vi "GrabberOPENandCLOSE.vi"(8 "Error In":errorcluster, 9 "Grabber Open/Close":bool, 11 "refnum name":string="My Solenoid RefNum") -> (0 "Error Out":errorcluster)   [LabVIEW 2014]
uses:
  <vilib>/Rock Robotics/WPI/Solenoid/WPI_SolenoidValue.ctl
  <vilib>/Rock Robotics/WPI/Solenoid/WPI_SolenoidSetEnum.vi
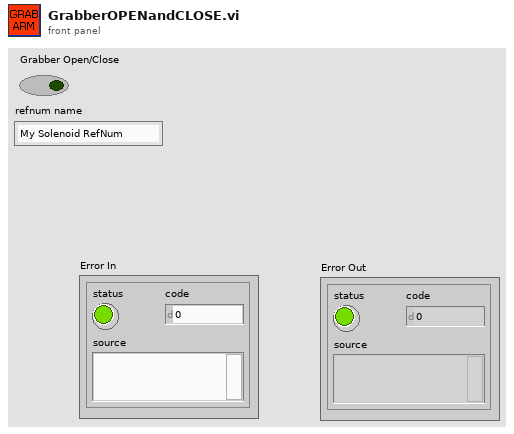
[diagram p1: front panel]
types:
  T1 = typedef "WPI_SolenoidValue.ctl" = enum16{"Off", "On", "Forward", "Reverse"}
  T2 = typedef "WPI_SolenoidDevRef.ctl" = cluster{"DevStatus":errorcluster, "Pneumatics Control Module":u8, "Forward Solenoid Channel":T3, "Reverse Solenoid Channel":T3}
  T3 = typedef "WPI_SolenoidChannel.ctl" = enum8{"Solenoid 0", "Solenoid 1", "Solenoid 2", "Solenoid 3", "Solenoid 4", "Solenoid 5", "Solenoid 6", "Solenoid 7", "Invalid"}
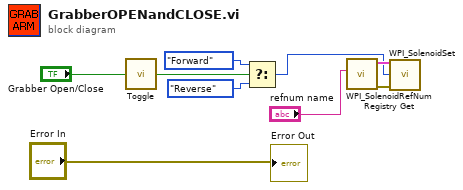
[diagram p0: block diagram]
diagram:
  n1 = call "Toggle.vi"("Input"="Grabber Open/Close") -> ("Output"=w9:bool)
  n2 = Select(t=WPI_SolenoidValue."Forward" ("Value"), s=w9, f=WPI_SolenoidValue."Reverse" ("Value")) -> (s? t:f=w4:T1)
  n3 = call <vilib>:"WPI_SolenoidRefNum Registry Get.vi"("refnum name"="refnum name") -> ("error out"=w6:errorcluster, "SolenoidDevRef"=w5:T2)  [unwired: 9 in]
  n4 = call-poly <vilib>:"WPI_SolenoidSet.vi"("error in (no error)"=w6, "Value"=w4, "SolenoidDevRef"=w5) -> ()  [unwired: 7 in, 2 out]
  "Error Out" <- "Error In"
